vi "Emerson 5700 Hot Density Calculation.vi"(7 "Water Properties Reference":T1, 8 "Error In":errorcluster, 11 "RTD Out (°F)":dbl format="%#.6g") -> (0 "Error Out":errorcluster, 3 "Density (lb/gal)":dbl format="%#.9g")   [LabVIEW 2020]
uses:
  HEWH Water Properties.ctl
panel:
  out "Upper/Lower":dbl format="%.15g"
  in  "CSA Alternate Data":string[][](array[string])=array1102x4[4408 elements]
  out "Upper6":dbl format="%#.6g"
  out "Upper5":dbl format="%#.6g"
  out "Upper4":dbl format="%#.6g"
  out "Upper3":dbl format="%#.6g"
  out "Upper2":dbl format="%#.6g"
  out "Upper1":dbl format="%#.6g"
  out "Lower":dbl format="%.7g"
  out "Upper":dbl format="%.7f"
  out "RTDK":dbl format="%.6g"
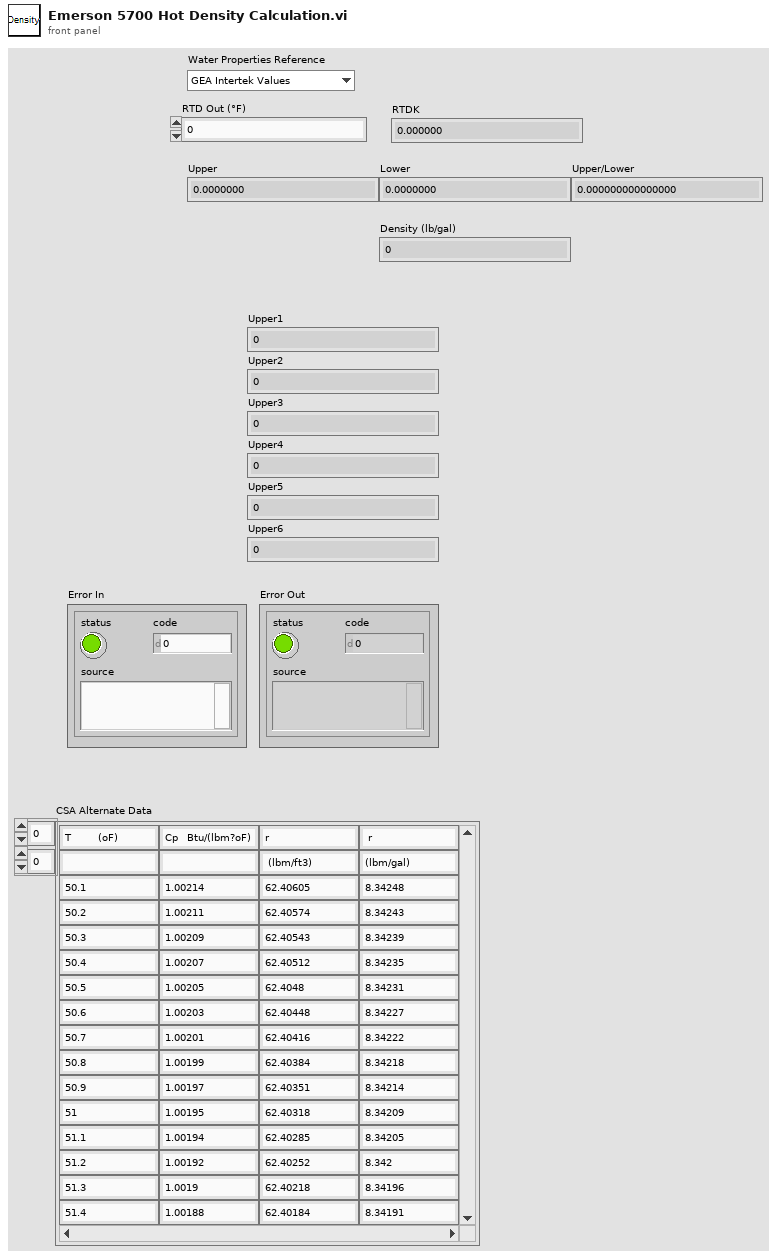
[diagram p1: front panel]
types:
  T1 = typedef "HEWH Water Properties.ctl" = enum16{"GEA Intertek Values", "CSA Values", "ANSI Values"}
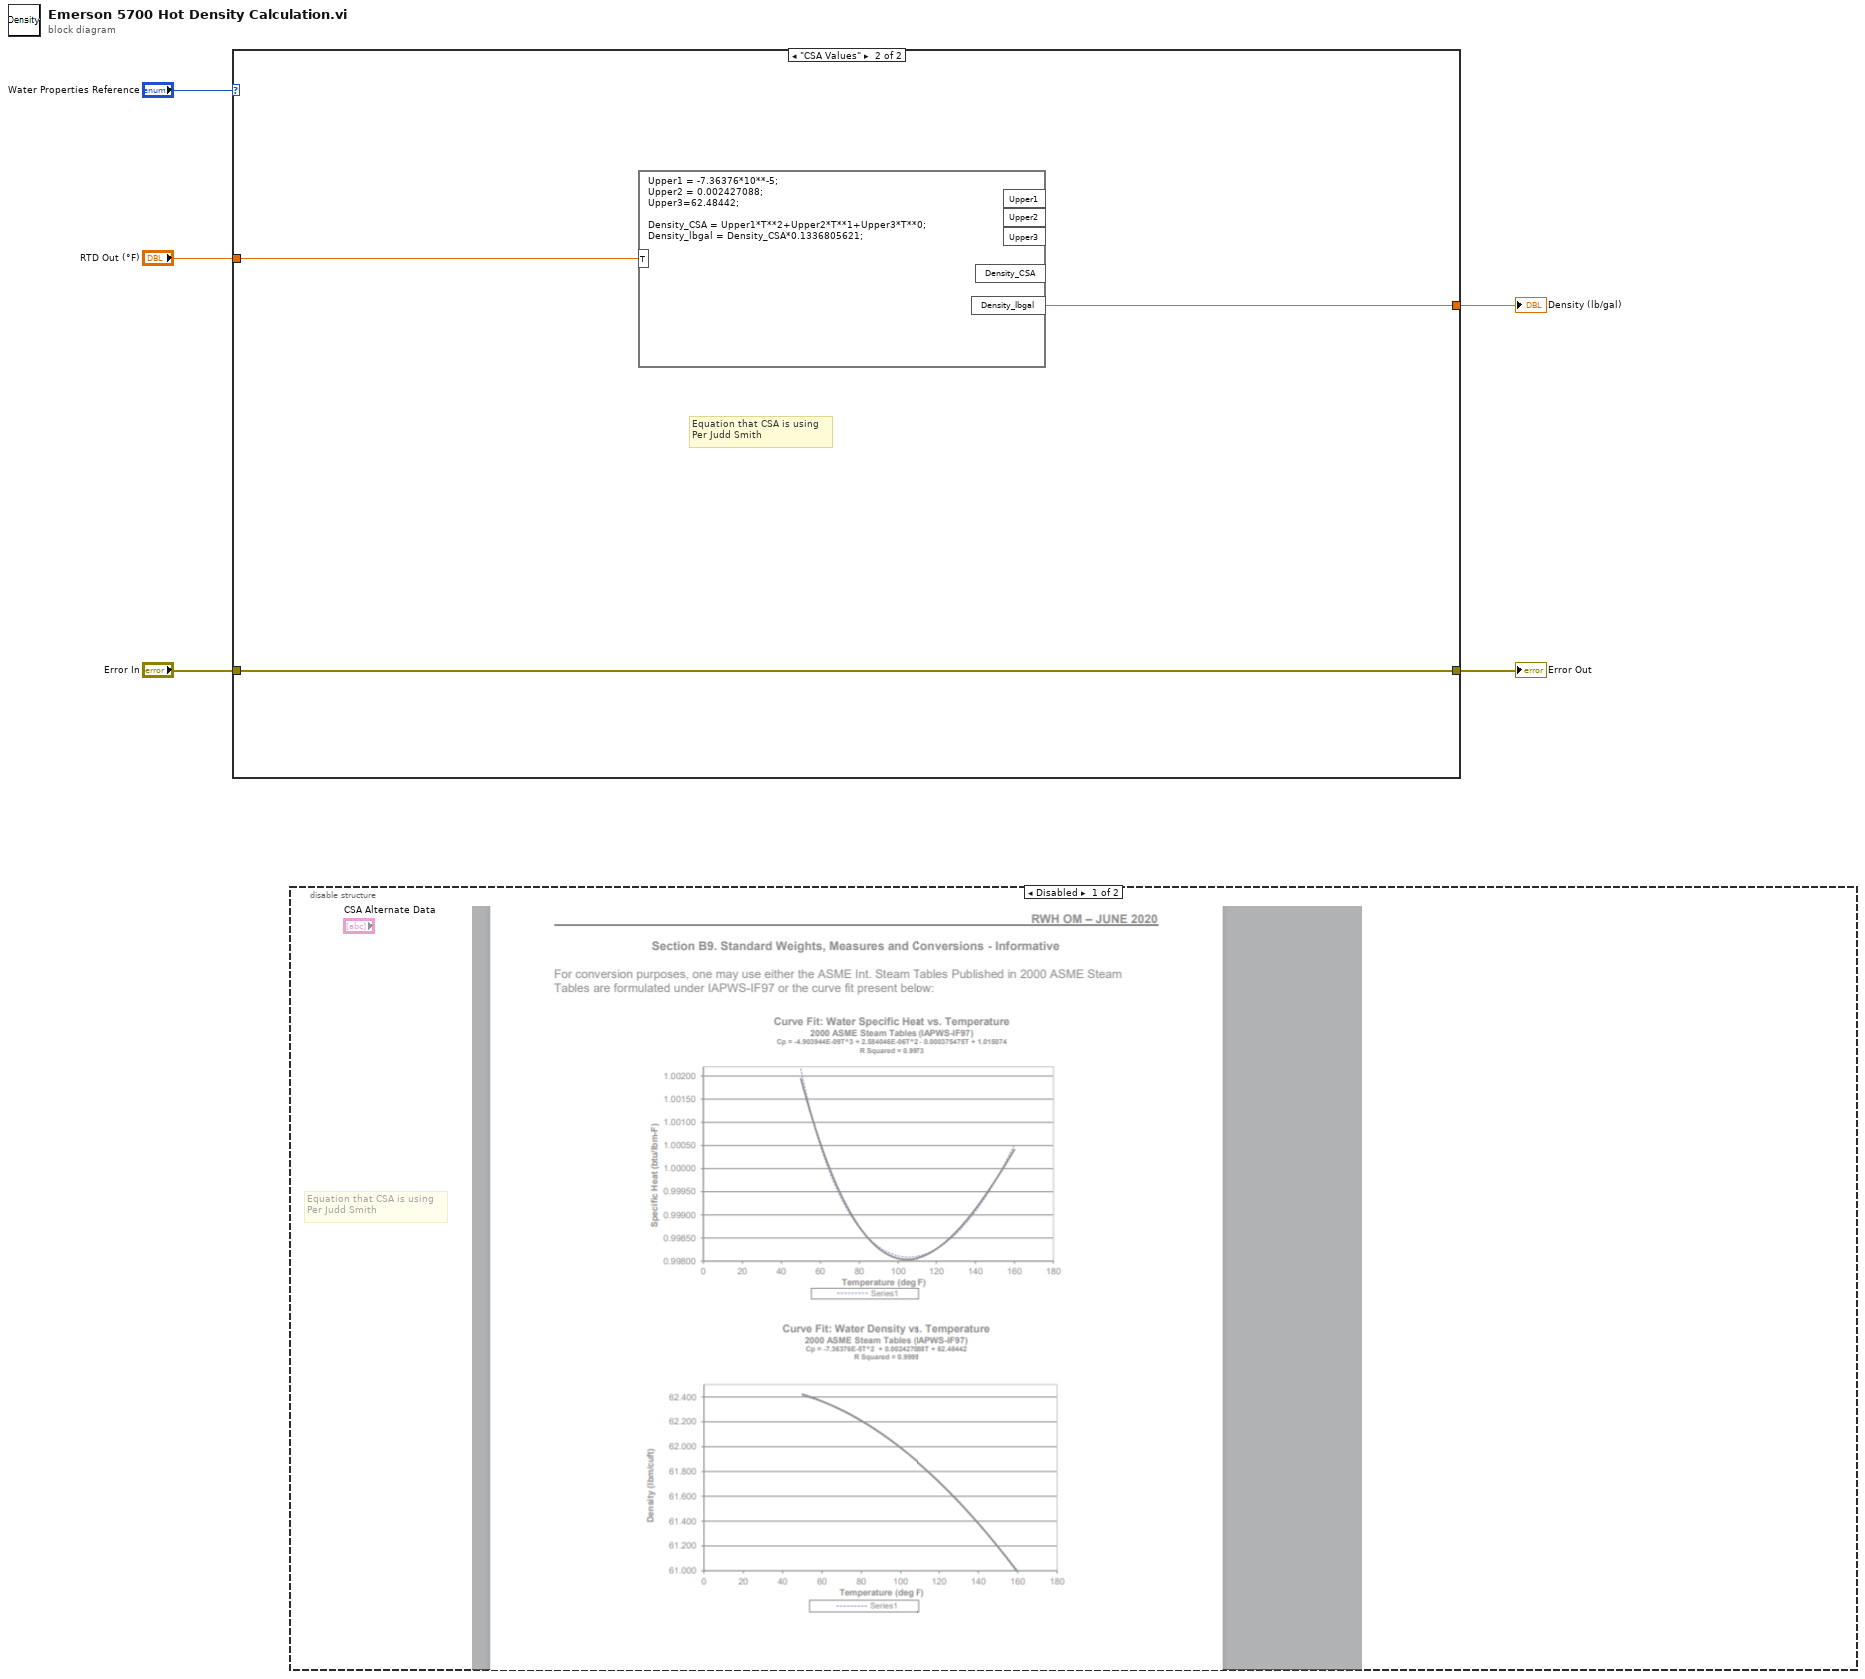
[diagram p0: block diagram]
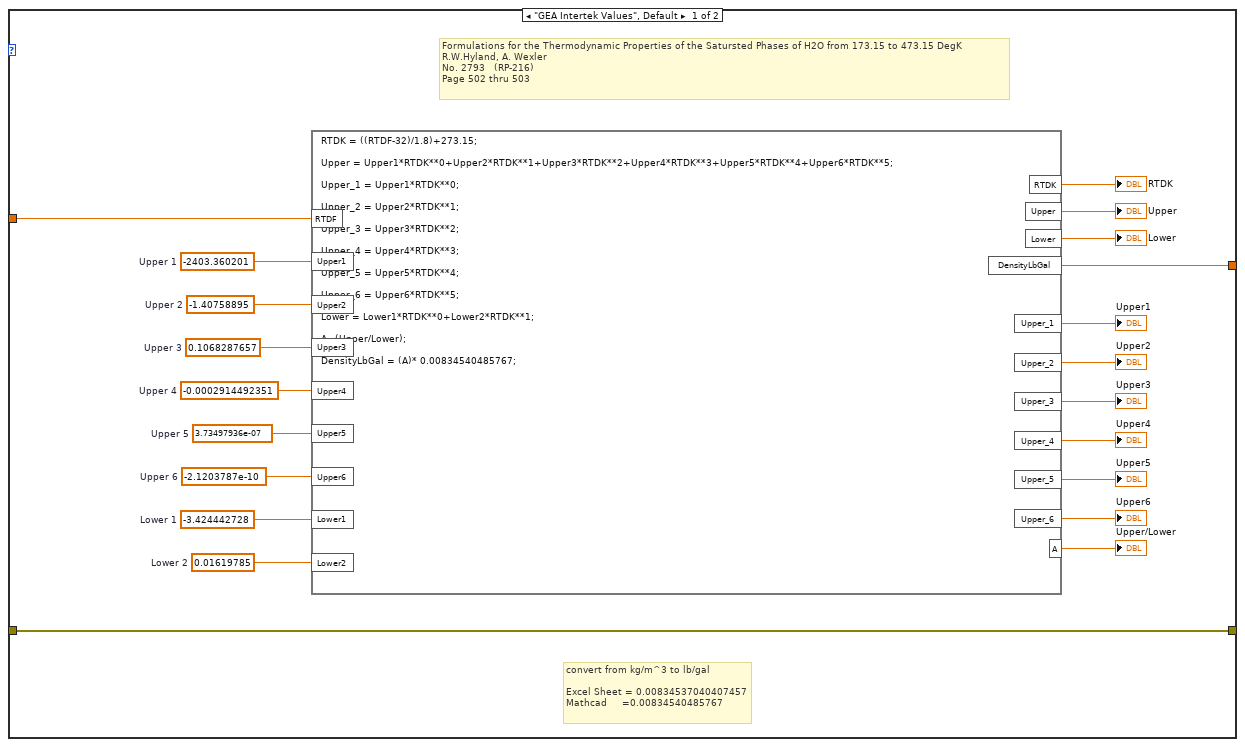
[diagram p2: hidden frame]
diagram:
  n1 = case shown="\"CSA Values\"" "Water Properties Reference" {
    tunnel: "RTD Out (°F)" -> [w26 w28]
    tunnel: [w14 w27] -> w4
    tunnel: "Error In" -> [w6 w29]
    tunnel: [w6 w29] -> w2
    frame "GEA Intertek Values", Default {
      w17 = 0.01619785  # Lower 2
      w16 = -3.424442728  # Lower 1
      w19 = -2.1203787e-10  # Upper 6
      w20 = 3.73497936e-07  # Upper 5
      w21 = -0.0002914492351  # Upper 4
      w22 = 0.1068287657  # Upper 3
      w23 = -1.40758895  # Upper 2
      w24 = -2403.360201  # Upper 1
      # "convert from kg/m^3 to lb/gal\n\nExcel Sheet = 0.00834537040407457\nMathcad     =0.00834540485767"
      # "Formulations for the Thermodynamic Properties of the Satursted Phases of H2O from 173.15 to 473.15 DegK\nR.W.Hyland, A. Wexler\nNo. 2793   (RP-216)\nPage 502 thru 503"
      n2 = formula code="RTDK = ((RTDF-32)/1.8)+273.15;\n\nUpper = Upper1*RTDK**0+Upper2*RTDK**1+Upper3*RTDK**2+Upper4*RTDK**3+Upper5*RTDK**4+Upper6*RTDK**5;\n\nUpper_1 = Upper1*RTDK**0;\n\nUpper_2 = Upper2*RTDK**1;\n\nUpper_3 = Upper3*RTDK**2;\n\nUpper_4 = Upper4*RTDK**3;\n\nUpper_5 = Upper5*RTDK**4;\n\nUpper_6 = Upper6*RTDK**5;\n\nLower = Lower1*RTDK**0+Lower2*RTDK**1;\n\nA=(Upper/Lower);\n\nDensityLbGal = (A)* 0.00834540485767;"("RTDF"=w26, "Upper1"=w24, "Upper2"=w23, "Upper3"=w22, "Upper4"=w21, "Upper5"=w20, "Upper6"=w19, "Lower1"=w16, "Lower2"=w17) -> ("RTDK"=→"RTDK":dbl, "Upper"=→"Upper":dbl, "Lower"=→"Lower":dbl, "DensityLbGal"=w14:dbl, "Upper_1"=→"Upper1":dbl, "Upper_2"=→"Upper2":dbl, "Upper_3"=→"Upper3":dbl, "Upper_4"=→"Upper4":dbl, "Upper_5"=→"Upper5":dbl, "Upper_6"=→"Upper6":dbl, "A"=→"Upper/Lower":dbl)
    }
    frame "CSA Values" {
      # "Equation that CSA is using\nPer Judd Smith"
      n3 = formula code="Upper1 = -7.36376*10**-5;\nUpper2 = 0.002427088;\nUpper3=62.48442;\n\nDensity_CSA = Upper1*T**2+Upper2*T**1+Upper3*T**0;\nDensity_lbgal = Density_CSA*0.1336805621;"("T"=w28) -> ("Density_lbgal"=w27:dbl)  [unwired: 4 out]
    }
  }
  "Error Out" <- w2
  "Density (lb/gal)" <- w4
  n4 = disable-structure shown="Disabled" {
    frame Disabled {
      # "Equation that CSA is using\nPer Judd Smith"
    }
    frame Enabled {
    }
  }
